vi "Errorbar2012.vi"   [LabVIEW 2013]
uses:
  <vilib>/Heliosphere Research LLC/Advanced Plotting Toolkit/api_plotting/ScatterProperties.ctl
  <vilib>/Heliosphere Research LLC/Advanced Plotting Toolkit/properties/Marker.ctl
  <vilib>/Heliosphere Research LLC/Advanced Plotting Toolkit/properties/Marker_Style.ctl
  <vilib>/Heliosphere Research LLC/Advanced Plotting Toolkit/typedefs/PlotColor.ctl
  <vilib>/Heliosphere Research LLC/Advanced Plotting Toolkit/properties/Line.ctl
  <vilib>/Heliosphere Research LLC/Advanced Plotting Toolkit/properties/Line_Style.ctl
  <vilib>/Heliosphere Research LLC/Advanced Plotting Toolkit/properties/Colormap.ctl
  <vilib>/Heliosphere Research LLC/Advanced Plotting Toolkit/properties/Colormap_Map.ctl
  <vilib>/Heliosphere Research LLC/Advanced Plotting Toolkit/properties/Colormap_Scaling.ctl
  <vilib>/Heliosphere Research LLC/Advanced Plotting Toolkit/properties/Display.ctl
  ModeType.ctl
  <vilib>/Heliosphere Research LLC/Advanced Plotting Toolkit/Advanced Plotting Toolkit.lvlib
types:
  T1 = typedef "ModeType.ctl" = enum16{"Normal", "Expected Failure", "Skipped", "Broken"}
  T2 = typedef "Advanced Plotting Toolkit.lvlib/PlotColor.ctl" = u32
  T3 = typedef "Advanced Plotting Toolkit.lvlib/ScatterProperties.ctl" = cluster{"Marker":T4, "Line":T6, "Colormap":T8, "Display":T11}
  T4 = typedef "Advanced Plotting Toolkit.lvlib/Marker.ctl" = cluster{"Style":T5, "Color":T2, "Size":dbl}
  T5 = typedef "Advanced Plotting Toolkit.lvlib/Marker_Style.ctl" = enum16{"Automatic", "Circle", "Square", "Triangle", "Diamond", "Star", "Invisible"}
  T6 = typedef "Advanced Plotting Toolkit.lvlib/Line.ctl" = cluster{"Style":T7, "Color":T2, "Width":sgl}
  T7 = typedef "Advanced Plotting Toolkit.lvlib/Line_Style.ctl" = enum16{"Automatic", "Solid", "Dashed", "Dotted", "Dash-dot", "Invisible"}
  T8 = typedef "Advanced Plotting Toolkit.lvlib/Colormap.ctl" = cluster{"Map":T9, "Value Min":dbl, "Value Max":dbl, "Scaling":T10, "Reverse":bool}
  T9 = typedef "Advanced Plotting Toolkit.lvlib/Colormap_Map.ctl" = enum16{"Automatic", "Rainbow", "Hot and Cold", "White-Black", "White-Blue", "White-Green", "White-Red", "Fire", "Water", "Earth", "Air", "Pastel", "Banded", "Stepped"}
  T10 = typedef "Advanced Plotting Toolkit.lvlib/Colormap_Scaling.ctl" = enum16{"Default"}
  T11 = typedef "Advanced Plotting Toolkit.lvlib/Display.ctl" = cluster{"Alpha":dbl, "Z Order":dbl}
  T12 = typedef "Advanced Plotting Toolkit.lvlib/PlotID.ctl" = i32
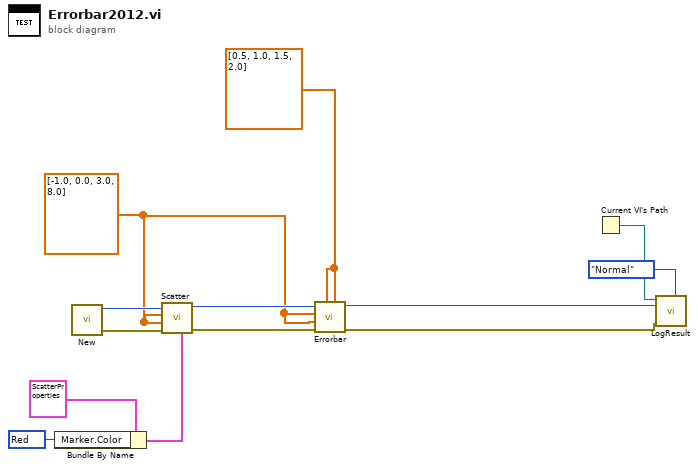
[diagram p0: block diagram]
diagram:
  w2 = T2 16711680 items=["Automatic"=2147483647, "Black"=0, "White"=16777215, "Red"=16711680, "Green"=2263842, "Blue"=255, "Cyan"=65535, "Magenta"=16711935, "Yellow"=16776960] ("Marker.Color")
  w5 = dbl[] [0.5, 1.0, 1.5, 2.0] ("X Errors")
  w6 = dbl[] [-1.0, 0.0, 3.0, 8.0] ("X Data")
  n1 = Bundle By Name(cluster=T3 {"Marker"={"Style"=enum."Automatic", "Color"=2147483647, "Size"=nan}, "Line"={"Style"=enum."Automatic", "Color"=2147483647, "Width"=nan}, "Colormap"={"Map"=enum."Automatic", "Value Min"=nan, "Value Max"=nan, "Scaling"=enum."Default", "Reverse"=FALSE}, "Display"={"Alpha"=nan, "Z Order"=nan}} ("Scatter Properties"), "Marker.Color"=w2) -> (w3:T3)
  n2 = call <vilib>:"New.vi"() -> ("error out"=w7:errorcluster, "Plot ID"=w10:T12)  [unwired: 10 in]
  n3 = call <vilib>:"Scatter.vi"("Properties"=w3, "error in (no error)"=w7, "Y Data"=w6, "X Data"=w6, "Plot ID"=w10) -> ("error out"=w8:errorcluster, "Plot ID Out"=w9:T12)  [unwired: 5 in]
  n4 = call <vilib>:"Errorbar.vi"("Y Errors"=w5, "X Errors"=w5, "error in (no error)"=w8, "Y Data"=w6, "X Data"=w6, "Plot ID"=w9) -> ("error out"=w11:errorcluster, "Plot ID out"=w12:T12)  [unwired: 4 in]
  n5 = Current VI's Path() -> (path=w13:path)
  n6 = call "LogResult.vi"("Mode"=ModeType."Normal", "Test Result"=w11, "Test Artifact"=w12, "VI Path"=w13) -> ()  [unwired: 8 in]
